vi "TestVI.vi"(7 "Cluster in":T1, 8 "error in":errorcluster, 9 "Limit":string, 10 "Describe":string, 11 "TestItem":T2=enum."idle") -> (0 "Error Out":errorcluster, 3 "Result\n0.Item\n1.data\n2.limit\n3.result":string[](array[string]), 5 "Cluster out":T1)   [LabVIEW 2013]
uses:
  TestItem.ctl
  MainProgram/Control/Buffer.vi
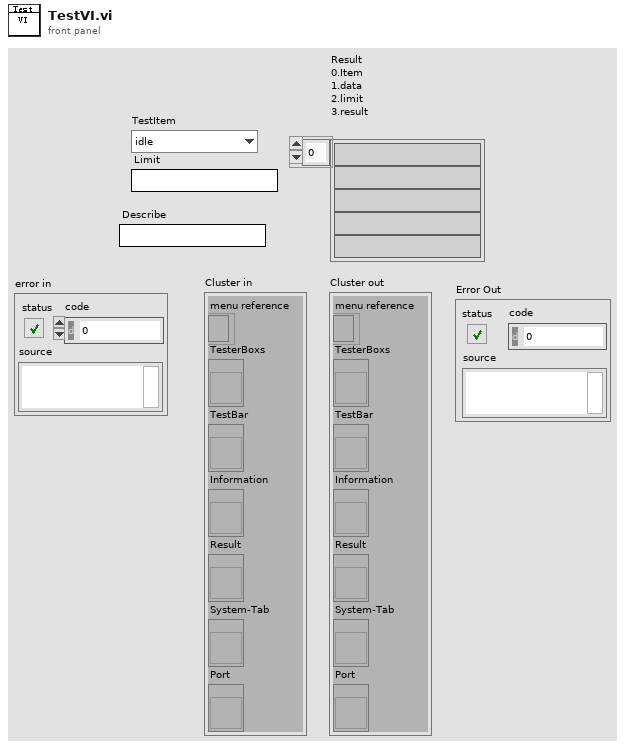
[diagram p1: front panel]
types:
  T1 = cluster{"menu reference":refnum<k9>, "TesterBoxs":refnum<vi>, "TestBar":refnum<vi>, "Information":refnum<vi>, "Result":refnum<vi>, "System-Tab":refnum<vi>, "Port":refnum<vi>}
  T2 = typedef "TestItem.ctl" = enum16{"Dynamic_call", "idle", "Dialog", "Check_SF", "Delay", "Reset_HiPot", "HV_Test", "GB_Test", "Instrument_Write&Read_HIPOT", "Hipot_ReadResult", "Hipot_Close", "CheckModel", "ScanTestStart", "ScanMultChannel_DCV", "ScanOneChannel_DCV", "Diplay_TestList"}
  T3 = typedef "Port.ctl" = cluster{"Multimeter":refnum<visa-resource-name>, "ACsource ":refnum<visa-resource-name>, "GEA":refnum<visa-resource-name>, "WT200":refnum<visa-resource-name>, "AutoScan":refnum<visa-resource-name>, "lines":tag, "MabeCOM":refnum<visa-resource-name>}
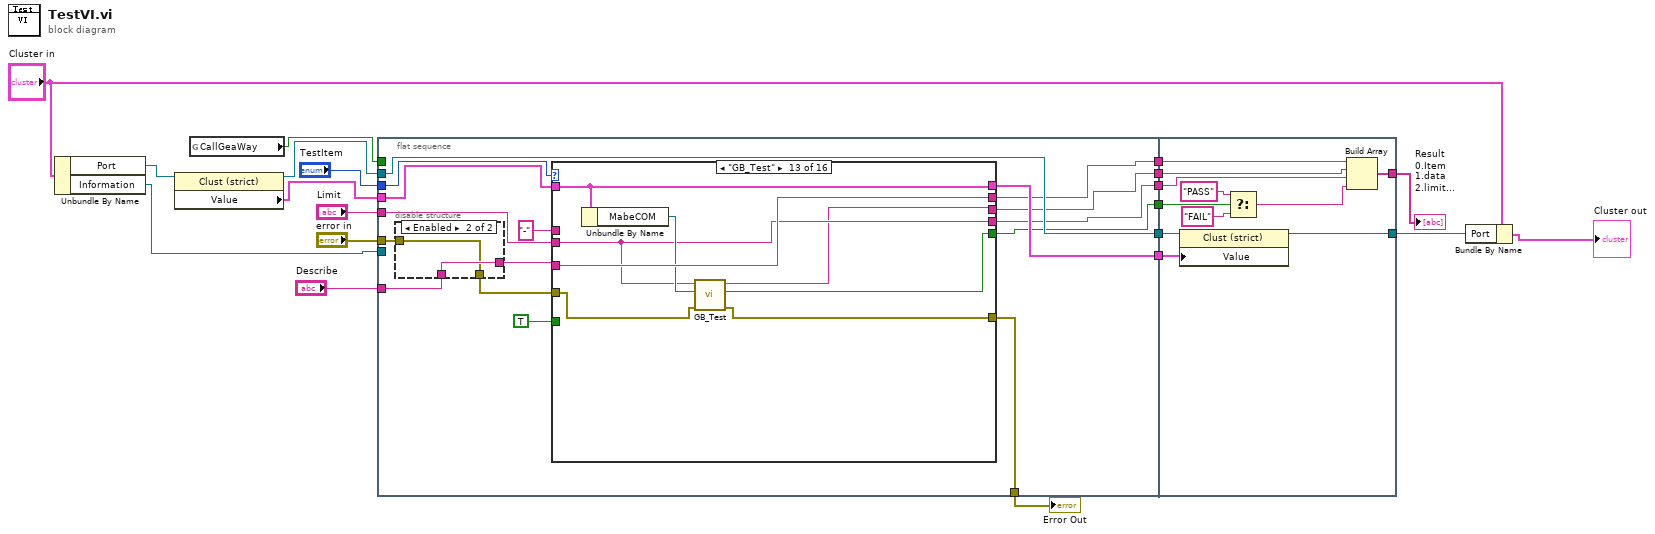
[diagram p0: block diagram]
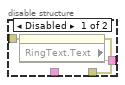
[diagram p2: hidden frame]
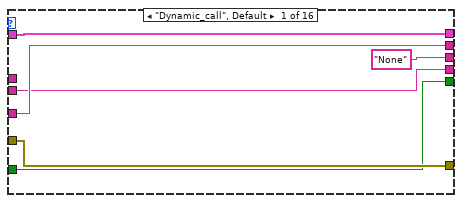
[diagram p3: hidden frame]
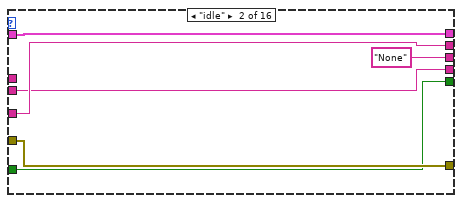
[diagram p4: hidden frame]
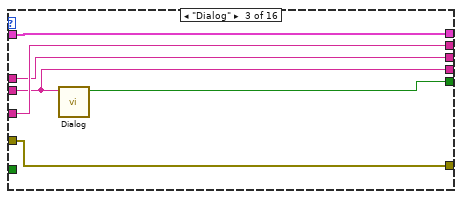
[diagram p5: hidden frame]
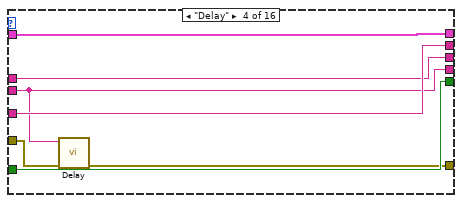
[diagram p6: hidden frame]
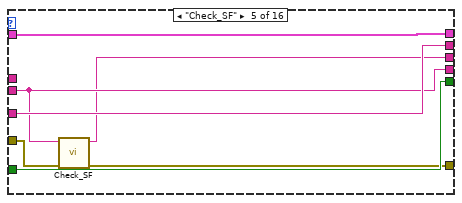
[diagram p7: hidden frame]
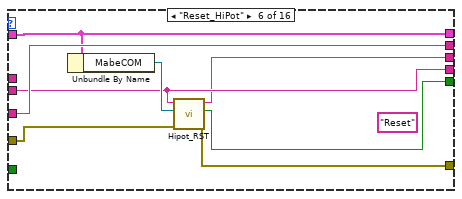
[diagram p8: hidden frame]
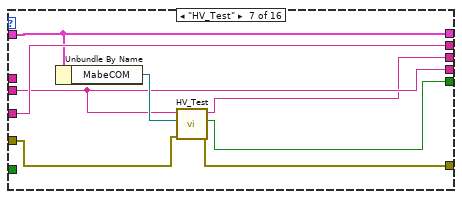
[diagram p9: hidden frame]
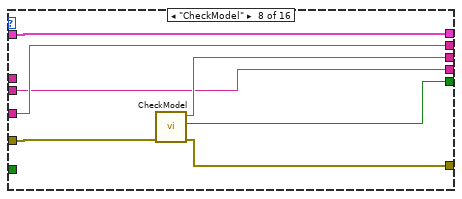
[diagram p10: hidden frame]
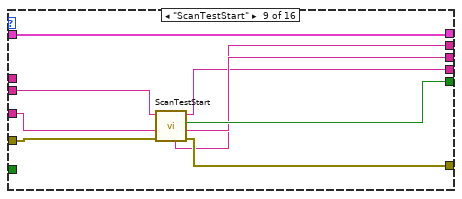
[diagram p11: hidden frame]
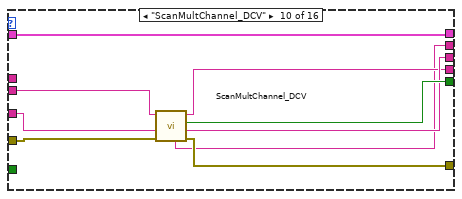
[diagram p12: hidden frame]
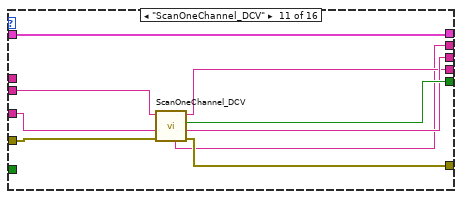
[diagram p13: hidden frame]
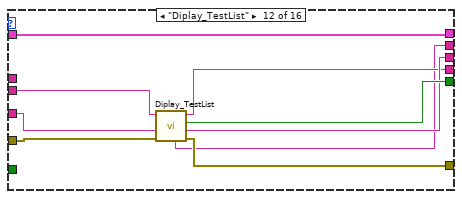
[diagram p14: hidden frame]
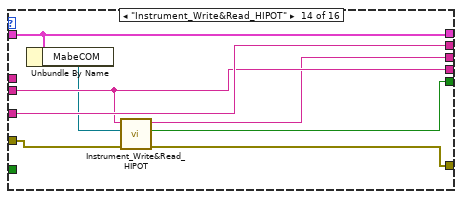
[diagram p15: hidden frame]
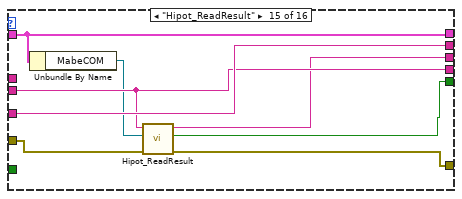
[diagram p16: hidden frame]
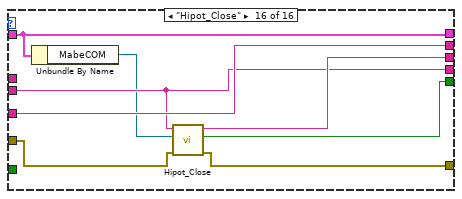
[diagram p17: hidden frame]
diagram:
  n1 = Unbundle By Name("Cluster in") -> ("Port"=w12:refnum<vi>, "Information"=w4:refnum<vi>)
  n2 = property class="Clust (strict)"(reference=w12) -> (reference out=w14:refnum<vi>, "Value"=w16:T3)  [unwired: 1 in, 1 out]
  n3 = global read "Buffer.vi" "CallGeaWay"() -> (w13:bool)
  n4 = flat-sequence {
    tunnel: "TestItem" -> [w35]
    tunnel: "Limit" -> [w32]
    tunnel: w16 -> [w34]
    tunnel: "error in" -> [w31]
    tunnel: [w36] -> w15
    tunnel: w14 -> [w36]
    tunnel: w13 -> [_]
    tunnel: w4 -> [_]
    tunnel: [w33] -> w10
    tunnel: [w29] -> w9
    tunnel: [w28] -> w8
    tunnel: [w27] -> w7
    tunnel: [w26] -> w6
    tunnel: [w25] -> w5
    tunnel: "Describe" -> [w21]
    tunnel: [w172] -> w17
    tunnel: w15 -> [w171]
    tunnel: [w170] -> w11
    tunnel: w10 -> [w169]
    tunnel: w8 -> [w168]
    tunnel: w7 -> [w167]
    tunnel: w6 -> [w166]
    tunnel: w5 -> [w165]
    frame #0 {
      n5 = disable-structure shown="Enabled" {
        disable-tunnel: w31 -> [w39 w40]
        disable-tunnel: [w38 w40] -> w30
        disable-tunnel: [w37 w41] -> w22
        disable-tunnel: w21 -> [_ w41]
        frame Disabled {
          n6 = property on="TestItem" class="Enum (strict)"(error in=w39) -> (error out=w38:errorcluster, "RingText.Text"=w37:string)  [unwired: 1 in, 1 out]
        }
        frame Enabled {
        }
      }
      n7 = case shown="\"GB_Test\"" w35 {
        tunnel: w34 -> [w47 w51 w58 w66 w73 w80 w85 w92 w97 w106 w115 w124 w136 w142 w151 w159]
        tunnel: [w47 w51 w58 w66 w73 w80 w85 w92 w97 w106 w115 w124 w136 w142 w151 w159] -> w33
        tunnel: w32 -> [w44 w50 w56 w62 w70 w78 w83 w91 w102 w111 w120 w129 w134 w147 w153 w160]
        tunnel: w30 -> [w46 w53 w55 w61 w69 w75 w87 w96 w105 w114 w123 w132 w138 w146 w155 w163]
        tunnel: [w46 w53 w55 w60 w68 w74 w86 w90 w103 w112 w121 w130 w137 w145 w154 w157] -> w29
        tunnel: [w42 w48 w57 w64 w71 w77 w88 w94 w104 w113 w122 w131 w139 w144 w149 w162] -> w28
        tunnel: ["None" ("TestData") "None" ("TestData") w54 w63 w67 w76 w82 w95 w101 w110 w119 w128 w133 w143 w152 w161] -> w27
        tunnel: [w44 w50 w56 w62 w70 w78 w83 w91 w100 w109 w118 w127 w134 w147 w153 w160] -> w26
        tunnel: [w45 w52 w59 w65 w72 w81 w89 w93 w98 w107 w116 w125 w140 w148 w156 w164] -> w25
        tunnel: w22 -> [w45 w52 w59 w65 w72 w81 w89 w93 w99 w108 w117 w126 w140 w148 w156 w164]
        tunnel: TRUE ("TestResult") -> [w42 w48 _ w64 w71 _ _ _ _ _ _ _ _ _ _ _]
        tunnel: "-" -> [_ _ w54 w63 _ _ _ _ _ _ _ _ _ _ _ _]
        frame "Dynamic_call", Default {
        }
        frame "idle" {
        }
        frame "Dialog" {
          n8 = call "Dialog.vi"("Limit"=w56) -> ("true"=w57:bool)  [unwired: 9 in, 1 out]
        }
        frame "Delay" {
          n9 = call "Delay.vi"("error in (no error)"=w61, "Limit"=w62) -> ("error out"=w60:errorcluster)  [unwired: 7 in, 2 out]
        }
        frame "Check_SF" {
          n10 = call "Check_SF.vi"("error in (no error)"=w69, "Limit"=w70) -> ("error out"=w68:errorcluster, "TestData"=w67:string)  [unwired: 7 in, 1 out]
        }
        frame "Reset_HiPot" {
          (unwired) "Reset"
          n11 = Unbundle By Name(w80) -> ("MabeCOM"=w79:refnum<visa-resource-name>)
          n12 = call "Hipot_RST.vi"("Error In"=w75, "PORT"=w79, "Limit"=w78) -> ("Error Out"=w74:errorcluster, "Result"=w77:bool, "Data"=w76:string)  [unwired: 6 in]
        }
        frame "HV_Test" {
          n13 = Unbundle By Name(w85) -> ("MabeCOM"=w84:refnum<visa-resource-name>)
          n14 = call "HV_Test.vi"("Error In"=w87, "PORT"=w84, "Limit"=w83) -> ("error out"=w86:errorcluster, "Result"=w88:bool, "Data"=w82:string)  [unwired: 6 in]
        }
        frame "CheckModel" {
          n15 = call "CheckModel.vi"("Error In"=w96) -> ("Error Out"=w90:errorcluster, "TestResult"=w94:bool, "TestData"=w95:string)  [unwired: 8 in]
        }
        frame "ScanTestStart" {
          n16 = call "ScanTestStart.vi"("error in (no error)"=w105, "Descripbe"=w99, "Limit input"=w102) -> ("error out"=w103:errorcluster, "TestData"=w101:string, "TestResult"=w104:bool, "Limit out"=w100:string, "Descripbe output"=w98:string)  [unwired: 3 in, 1 out]
        }
        frame "ScanMultChannel_DCV" {
          n17 = call "ScanMultChannel_DCV.vi"("error in (no error)"=w114, "Descripbe"=w108, "Limit input"=w111) -> ("error out"=w112:errorcluster, "TestData"=w110:string, "TestResult"=w113:bool, "Limit out"=w109:string, "Descripbe output"=w107:string)  [unwired: 3 in, 1 out]
        }
        frame "ScanOneChannel_DCV" {
          n18 = call "ScanOneChannel_DCV.vi"("error in (no error)"=w123, "Descripbe"=w117, "Limit input"=w120) -> ("error out"=w121:errorcluster, "TestData"=w119:string, "TestResult"=w122:bool, "Limit out"=w118:string, "Descripbe output"=w116:string)  [unwired: 3 in, 1 out]
        }
        frame "Diplay_TestList" {
          n19 = call "Diplay_TestList.vi"("error in (no error)"=w132, "Descripbe"=w126, "Limit input"=w129) -> ("error out"=w130:errorcluster, "TestData"=w128:string, "TestResult"=w131:bool, "Limit out"=w127:string, "Descripbe output"=w125:string)  [unwired: 4 in]
        }
        frame "GB_Test" {
          n20 = Unbundle By Name(w136) -> ("MabeCOM"=w135:refnum<visa-resource-name>)
          n21 = call "GB_Test.vi"("Error In"=w138, "PORT"=w135, "Limit"=w134) -> ("error out"=w137:errorcluster, "Result"=w139:bool, "Data"=w133:string)  [unwired: 6 in]
        }
        frame "Instrument_Write&Read_HIPOT" {
          n22 = Unbundle By Name(w142) -> ("MabeCOM"=w141:refnum<visa-resource-name>)
          n23 = call "Instrument_Write&Read_HIPOT.vi"("Error In"=w146, "PORT"=w141, "Limit"=w147) -> ("error out"=w145:errorcluster, "Result"=w144:bool, "Data"=w143:string)  [unwired: 6 in]
        }
        frame "Hipot_ReadResult" {
          n24 = Unbundle By Name(w151) -> ("MabeCOM"=w150:refnum<visa-resource-name>)
          n25 = call "Hipot_ReadResult.vi"("Error In"=w155, "PORT"=w150, "Limit"=w153) -> ("Error Out"=w154:errorcluster, "Result"=w149:bool, "Data"=w152:string)  [unwired: 6 in]
        }
        frame "Hipot_Close" {
          n26 = Unbundle By Name(w159) -> ("MabeCOM"=w158:refnum<visa-resource-name>)
          n27 = call "Hipot_Close.vi"("Error In"=w163, "PORT"=w158, "Limit"=w160) -> ("error out"=w157:errorcluster, "Result"=w162:bool, "Data"=w161:string)  [unwired: 6 in]
        }
      }
    }
    frame #1 {
      n28 = property class="Clust (strict)"(reference=w171, "Value"=w169) -> (reference out=w170:refnum<vi>)  [unwired: 1 in, 1 out]
      n29 = Select(t="PASS", s=w168, f="FAIL") -> (s? t:f=w173:string)
      n30 = Build Array(w165, w167, w166, w173) -> (w172:string[])
    }
  }
  n31 = Bundle By Name(cluster="Cluster in", "Port"=w11) -> (→"Cluster out":T1)
  "Result\n0.Item\n1.data\n2.limit\n3.result" <- w17
  "Error Out" <- w9
